vi "Timer_When_Start.vi"() -> ()   [LabVIEW 2018]
panel:
  in  "stop":bool
  in  "Reset":bool
  out "Time (sec))":dbl
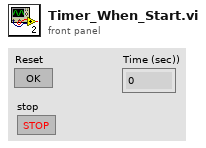
[diagram p1: front panel]
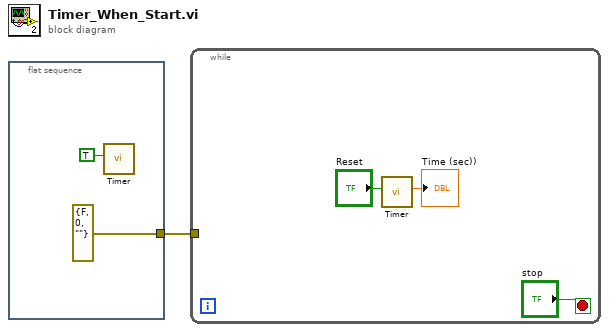
[diagram p0: block diagram]
diagram:
  n1 = flat-sequence {
    tunnel: [errorcluster {"status"=FALSE, "code"=0, "source"=""} ("error constant")] -> w1
    frame #0 {
      n2 = call "Timer.vi"("Reset"=TRUE) -> ()  [unwired: 10 in, 1 out]
    }
  }
  n3 = while {
    tunnel: w1 -> [_]
    stop <- "stop" stop-if-true
    n4 = call "Timer.vi"("Reset"="Reset") -> ("Time (sec))"=→"Time (sec))":dbl)  [unwired: 10 in]
  }
